vi "Write Environment Variable.vi"(8 "error in":errorcluster, 10 "value":string, 11 "name":string) -> (0 "error out":errorcluster)   [LabVIEW 2021, in "MeasurementServerTests.lvlib"]
uses:
  MeasurementServerTests.lvlib
  kernel32.dll
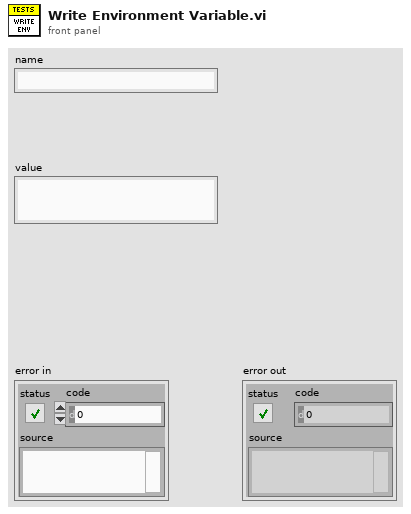
[diagram p1: front panel]
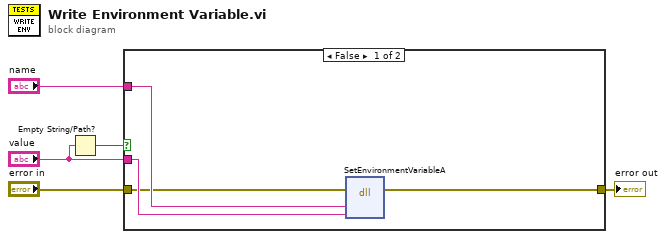
[diagram p0: block diagram]
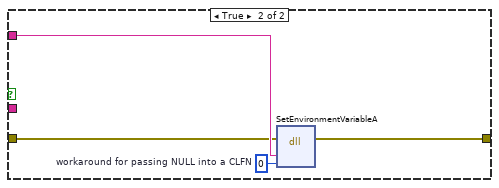
[diagram p2: hidden frame]
diagram:
  n1 = Empty String/Path?(string/path="value") -> (empty?=w5:bool)
  n2 = case shown="False" w5 {
    tunnel: "error in" -> [w7 w10]
    tunnel: "name" -> [w9 w11]
    tunnel: "value" -> [w8 _]
    tunnel: [w6 w12] -> w1
    frame False {
      n3 = dll-call lib="kernel32.dll" fn="SetEnvironmentVariableA"(error in=w7, "varName"=w9, "varValue"=w8) -> (error out=w6:errorcluster)  [unwired: 5 in, 1 out]
    }
    frame True {
      w13 = u64 0  # workaround for passing NULL into a CLFN
      n4 = dll-call lib="kernel32.dll" fn="SetEnvironmentVariableA"(error in=w10, "varName"=w11, "varValue"=w13) -> (error out=w12:errorcluster)  [unwired: 5 in, 1 out]
    }
  }
  "error out" <- w1
